vi "ATE_ops_cal_2.vi"() -> ()   [LabVIEW 2009]
doc: "Use this template to build a producer/consumer design pattern with events to produce queue items. Use this design pattern instead of the User Interface Event Handler pattern for user interfaces when you want to execute code asynchronously in response to an event without slowing the user interface responsiveness."
uses:
  Rvp8PowerData.ctl
  <vilib>/Analysis/NI_AALBase.lvlib
  <vilib>/Analysis/NI_AALPro.lvlib
panel:
  in  "ABORT":bool
  in  "READY":bool
  out "Instructions":string="rvp8 calibration vi\n\n1 - Disable or turn off transmitter\n2 - Stow Antenna (point vertically)\n3 - Start the labview program by clicking the Run arrow\n     (left most button under  drop down menues)\n     start cycle time about 35 seconds\n3 - Wait for the red 'BUSY' light to change to green 'READY'\n     The 'active' controls on the control tab are the 'TsPring/TsGrabber'\n     and the 'Start dBm', 'Step Size' and 'Steps' controls \n4 - Calibrate with the red  'Calibrate' button\n      calibration cycle time is about 5 minutes\n5 - Calibration cycle can be aborted with the 'Abort Cal' button which\n     is visable only during the cal cycle\n6 - exit the program with the red 'EXIT' button\n      exit cycle time about 20 seconds\n\nHints:\nWait for the green 'READY' light before clicking buttons"
  out "70dB\nAttenuators":bool[](array[boolean])
  out "70 Verfied":bool
  out "121dB\nAttenuators":bool[](array[boolean])
  out "121 Verified":bool
  in  "Configuration 1":bool
  out "Cal Output File":path
  out "Cal differences":cluster{dbl[], dbl[]}[](graph)
  out "RVP8 calibration":cluster{dbl[], dbl[]}[](graph)
  out "Cal file name":string
  in  "Cal data directory":string="/home/operator/ate/data/rvp8_cal"
  in  "Set SigGen":bool
  in  "Initialize":bool
  in  "70 dB":bool
  in  "121 dB":bool
  in  "Switches":bool
  in  "Calibrate":bool
  in  "Stop":bool
  in  "ATE TABS":enum32{"Status", "Controls"}(tab)=enum."Controls"
  out "ATE Switch Status":T1
  out "RVP8 Power":T2 {"time" format="%<%H:%M:%S\n%Y/%m/%d>T"}
  out "Signal Generator Status":T3={"Frequency (GHz)"=0.0, "RF Power (dBm)"=0.0, "RF Power"=TRUE} {"RF Power (dBm)" format="%.2g"}
  in  "Signal Generator Control":T4={"Frequency (GHz)"=2.809, "RF Power (dBm)"=-120.0, "RF ON/OFF"=FALSE}
  in  "Start dBm":dbl=-14.0 min=-100.0 max=14.0 step=1.0
  in  "Steps":i32=64
  in  "Steps Size":dbl=2.0 min=0.1 max=10.0 step=0.1 format="%.1g"
  in  "121 dB Atten":i32=121 min=0 max=121 step=1
  in  "70 dB Attn":i32=70 min=0 max=70 step=10
  in  "ATE Switches":T5={"Reversing Switch"=enum."Normal Function", "IO Switch #1 Input"=enum."NONE", "IO Switch #1 Output"=enum."NONE", "IO Switch #2 Input"=enum."NONE", "IO Switch #2 Output"=enum."NONE", "Signal Out Input"=enum."NONE", "Signal Out Output"=enum."NONE", "Signal Source Input"=enum."NONE", "Signal Source Output"=enum."NONE", "Power Meter Switch Input"=enum."NONE", "Pouer Meter Switch Output"=enum."NONE", "Amplifier Switch"=enum."Include Amp"}
  in  "DataSource":bool=TRUE
  out "P-State":string
  out "C-State":string
  in  "BUSY":bool
  # "ATE ops cal Program-II"
  # "10 dB"
  # "20 dB"
  # "40 dB"
  # "1 dB"
  # "2 dB"
  # "4 dB"
  # "4 dB"
  # "10 dB"
  # "20 dB"
  # "40 dB"
  # "40 dB"
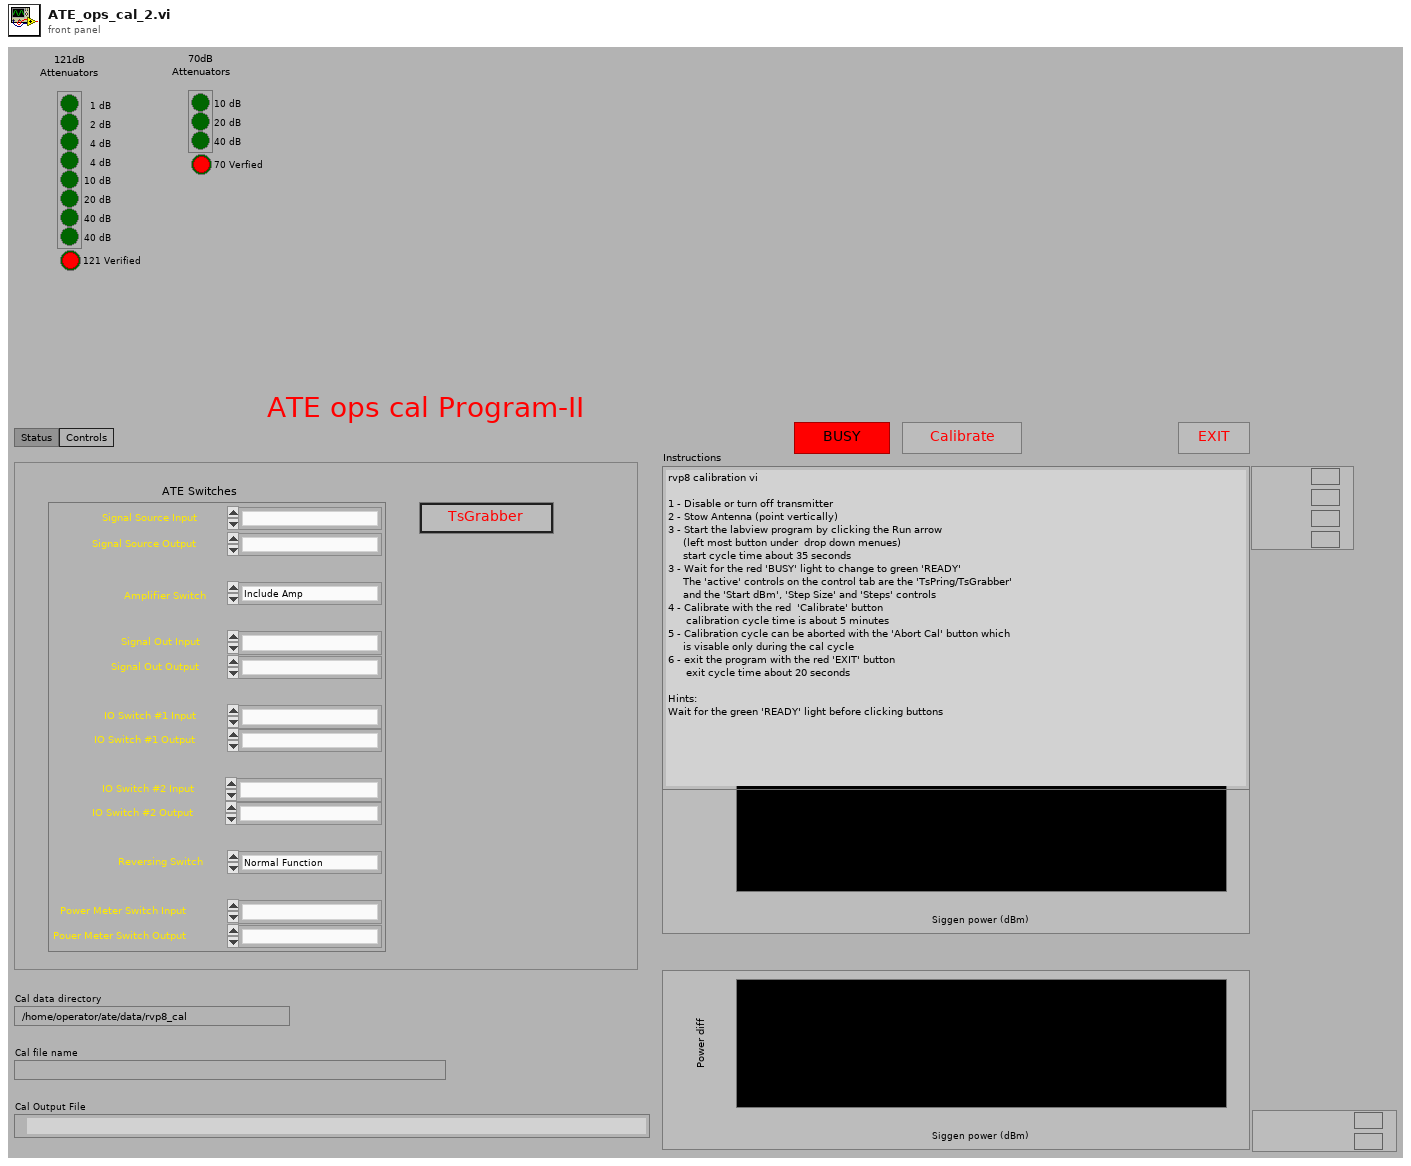
[diagram p1: front panel]
types:
  T1 = cluster{"Reversing Switch ":bool, "IO Switch #1":bool, "IO Switch #2":bool, "Signal Out":bool, "Signal Source":bool, "Power Meter":bool, "Amp By Pass":bool}
  T2 = typedef "Rvp8PowerData.ctl" = cluster{"success":bool, "time":dbl, "el":dbl, "az":dbl, "dbm0":dbl, "dbm1":dbl, "dbmHc":dbl, "dbmHx":dbl, "dbmVc":dbl, "dbmVx":dbl}
  T3 = cluster{"Frequency (GHz)":dbl, "RF Power (dBm)":dbl, "RF Power":bool}
  T4 = cluster{"Frequency (GHz)":dbl, "RF Power (dBm)":dbl, "RF ON/OFF":bool}
  T5 = cluster{"Reversing Switch":enum16{"Normal Function", "Reversing Function"}, "IO Switch #1 Input":enum16{"NONE", "AHR (J2)", "Splitter", "Signal Out Switch (S3)", "Reversing Switch"}, "IO Switch #1 Output":enum16{"NONE", "AHR (J2)", "Delay Device (S4)", "Power Meter Switch (S5)", "Reversing Switch"}, "IO Switch #2 Input":enum16{"NONE", "AVR (J3)", "Splitter", "Signal Out Switch (S3)", " 2W Term (TM1)", "Reversing Switch"}, "IO Switch #2 Output":enum16{"NONE", "AVR (J3)", "Signal Out Switch (S3)", "Power Meter Switch (S5)", "Reversing Switch", "2W Term (TM1)"}, "Signal Out Input":enum16{"NONE", "Amp Bypass Switch (S6)", "IO Switch #1 (S1)", "IO Switch #2 (S2)", "2W Term (TM3)"}, "Signal Out Output":enum16{"NONE", "2 Watt Term (TM3)", "Splitter", "Power Meter Switch (S5)"}, "Signal Source Input":enum16{"NONE", "Delay Device", "Signal Generator (J7)", "Inside Noise Box NF (J5)", "2W Term (TM3)"}, "Signal Source Output":enum16{"NONE", "Amp Bypass Switch", "Test Pulse Generator", "Power Meter Switch (S5)"}, "Power Meter Switch Input":enum16{"NONE", "IO Switch #1 (S1)", "Signal Source Switch (S4)", "Signal Out Switch (S3)", "IO Switch #2 (S2)", "TXH-TXV Switch (J8)"}, "Pouer Meter Switch Output":enum16{"NONE", "Power Meter (J6)"}, "Amplifier Switch":enum16{"Bypass Amp", "Include Amp"}}
  T6 = enum16{"open", "replace", "create", "open or create", "replace or create", "replace or create with confirmation"}
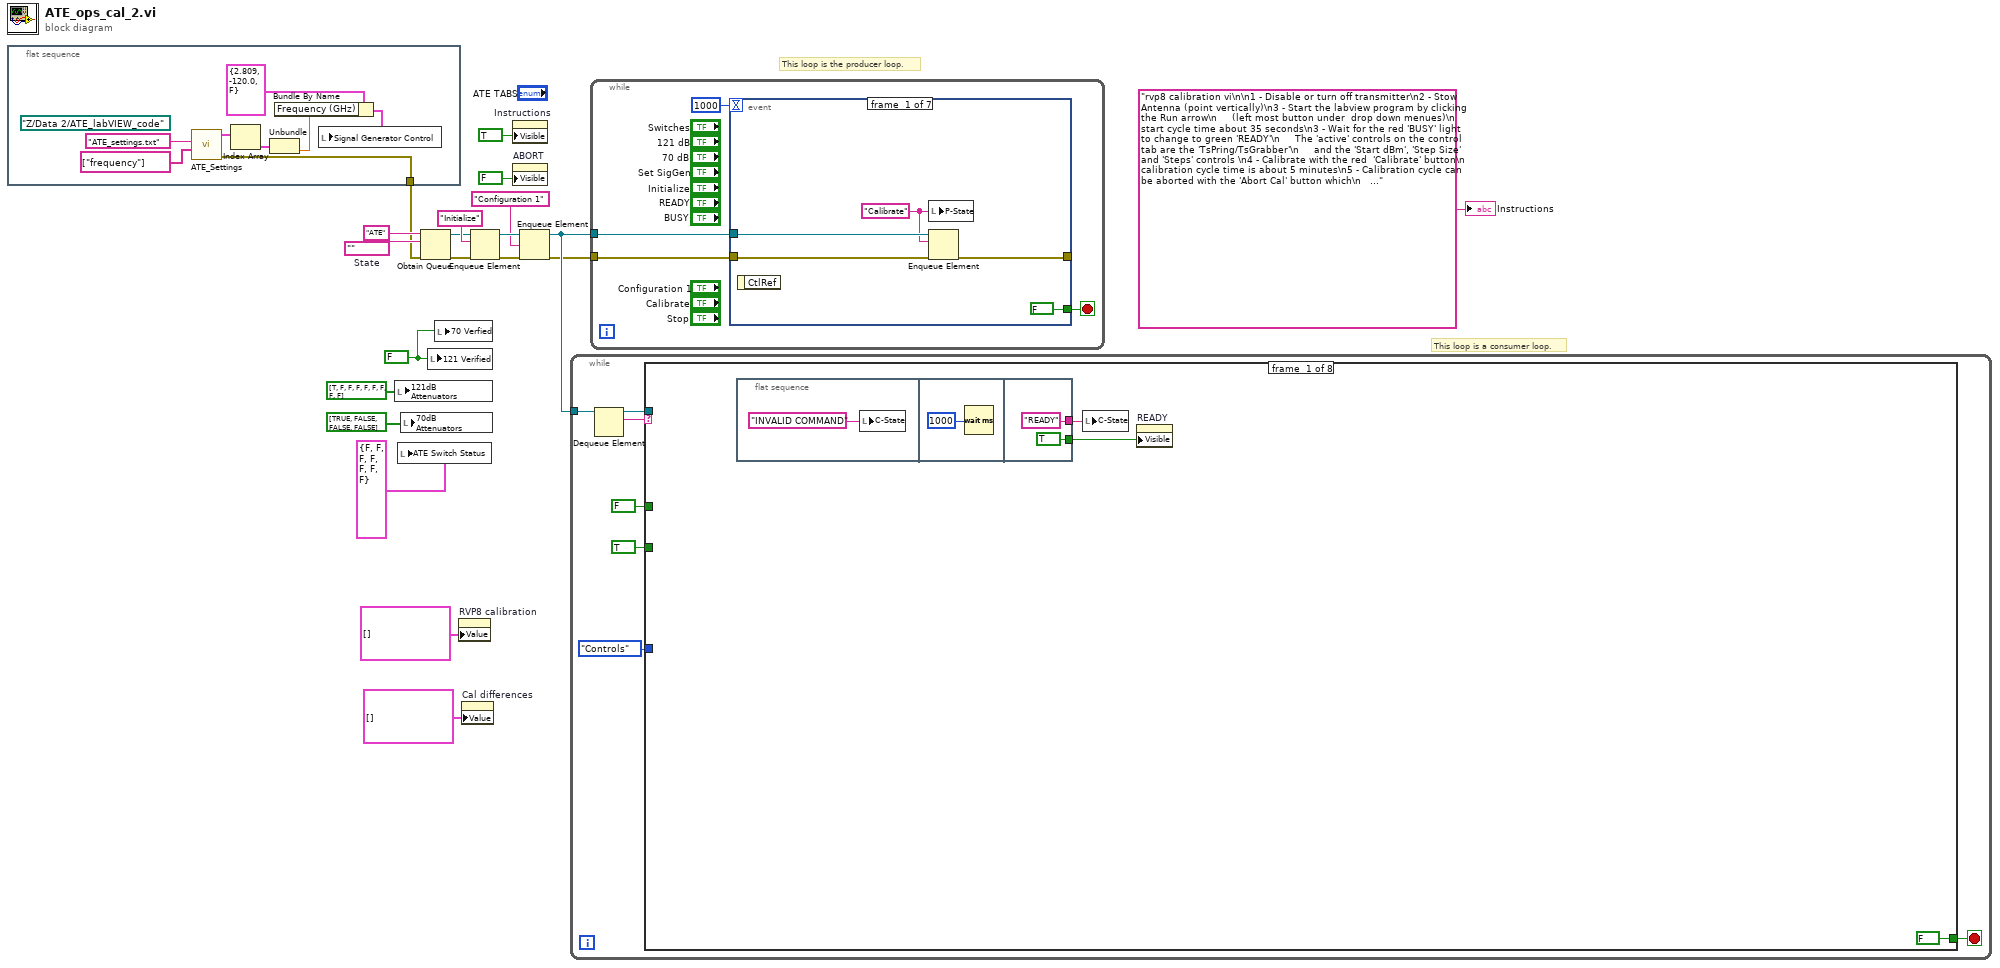
[diagram p0: block diagram]
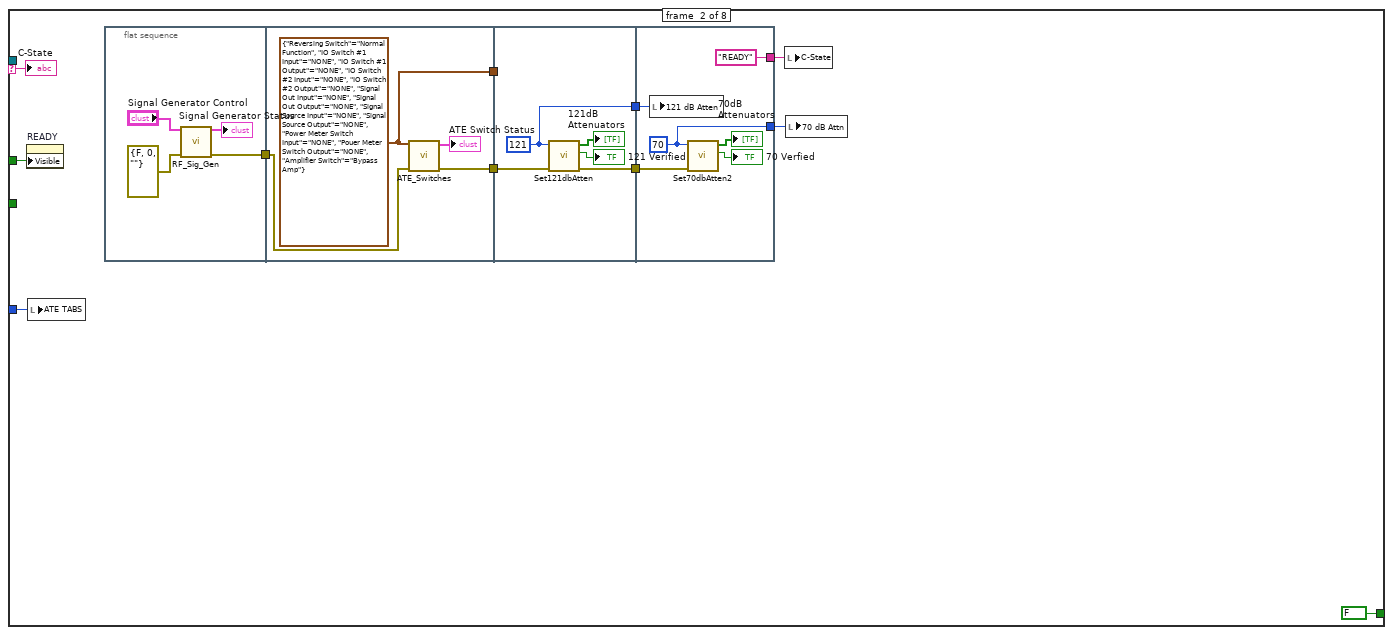
[diagram p2: hidden frame]
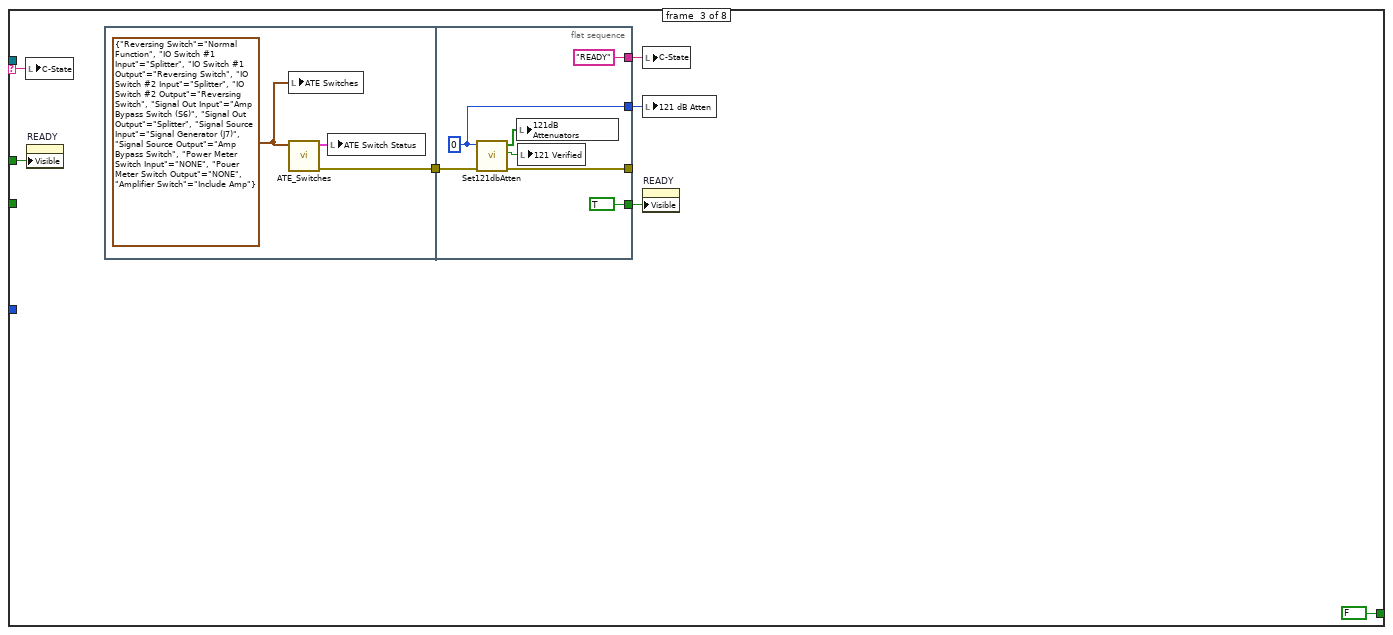
[diagram p3: hidden frame]
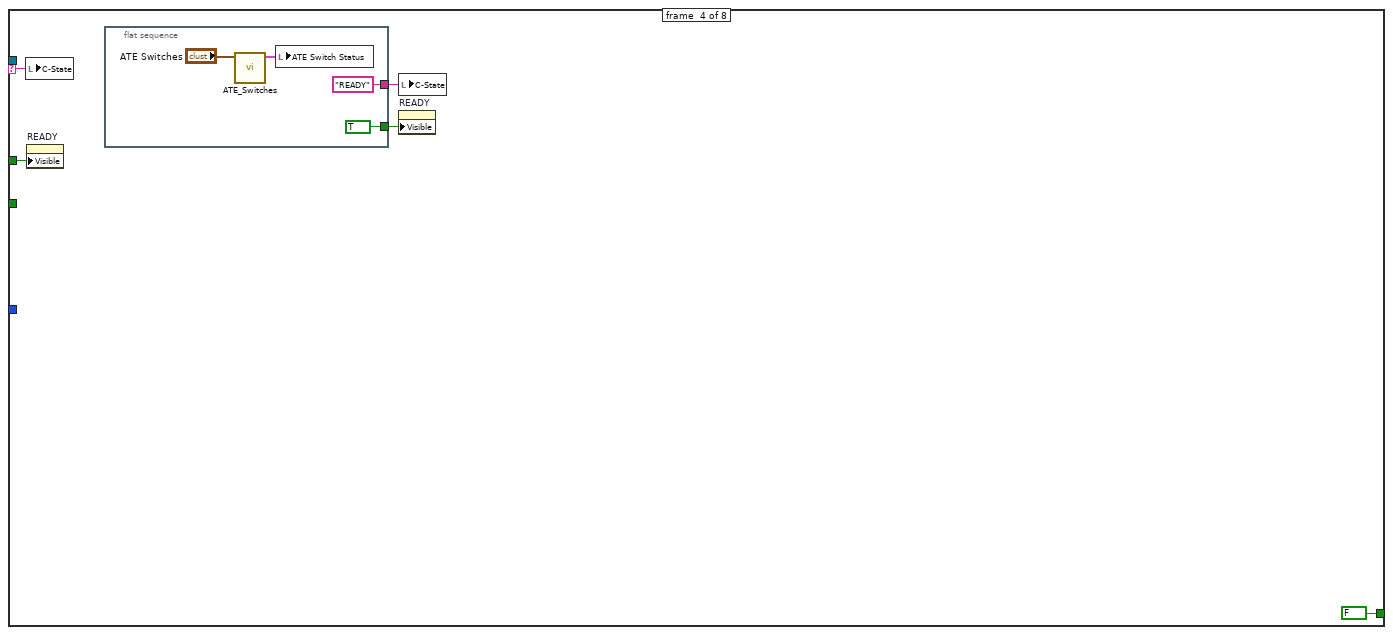
[diagram p4: hidden frame]
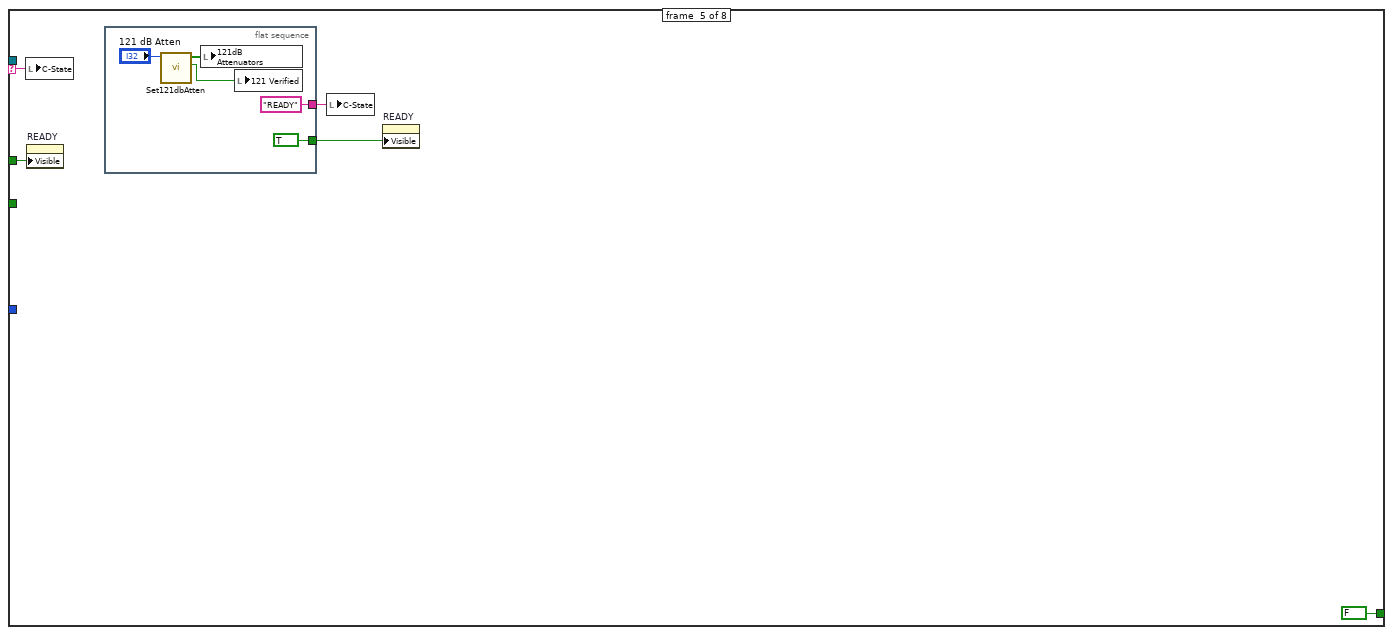
[diagram p5: hidden frame]
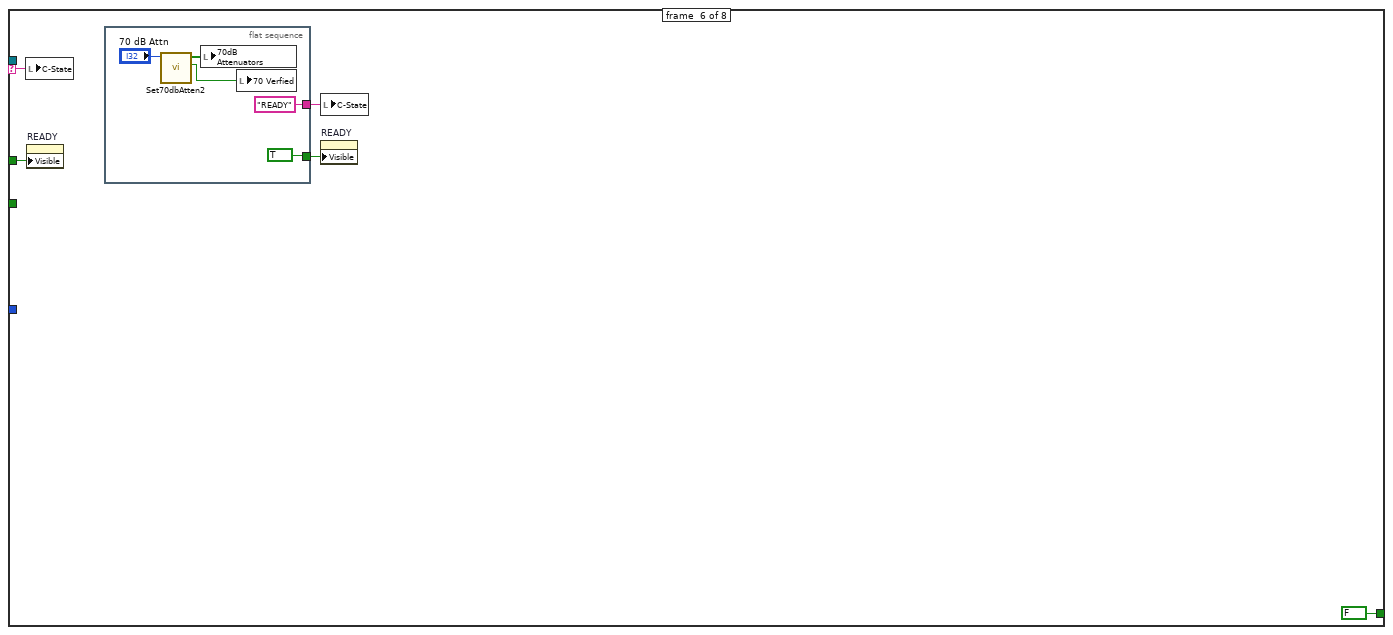
[diagram p6: hidden frame]
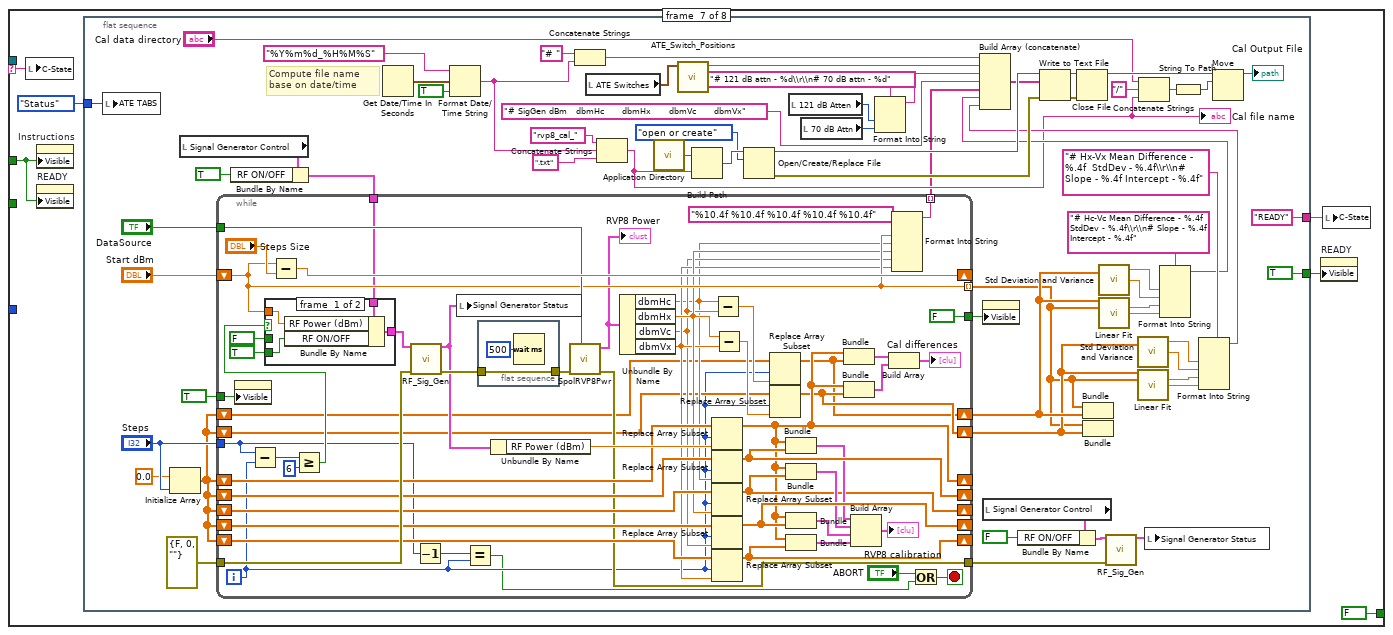
[diagram p7: hidden frame]
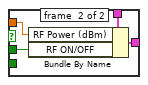
[diagram p8: hidden frame]
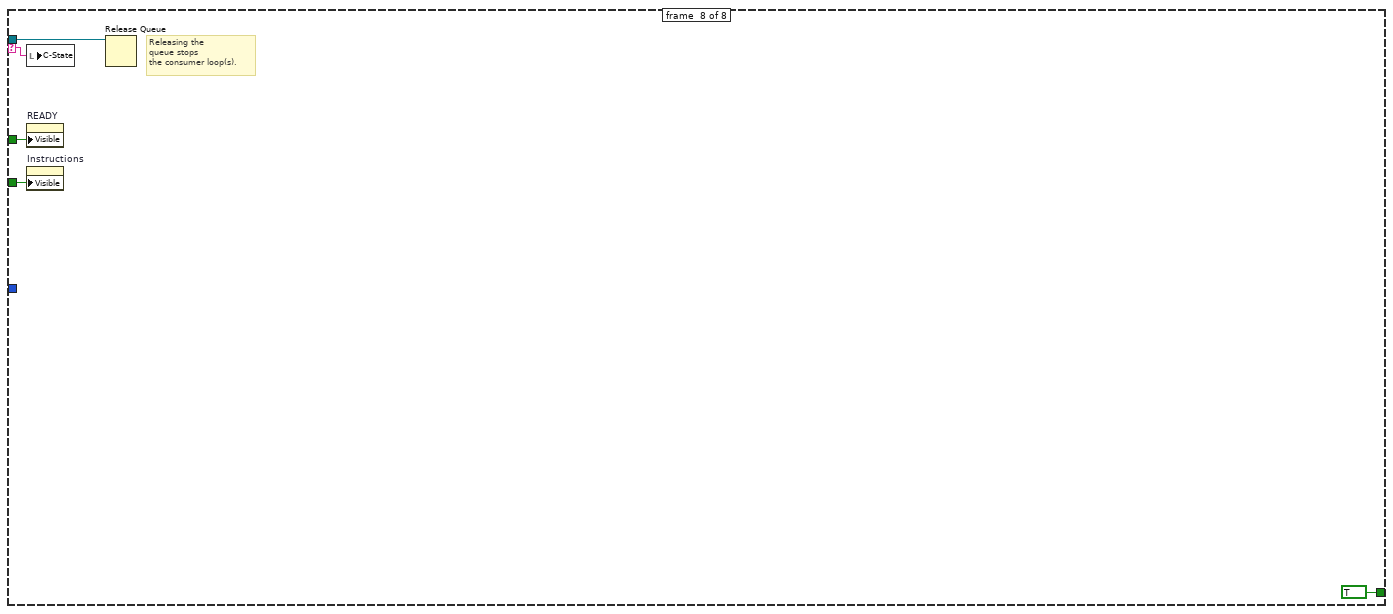
[diagram p9: hidden frame]
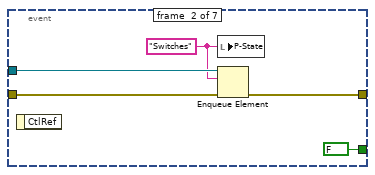
[diagram p10: hidden frame]
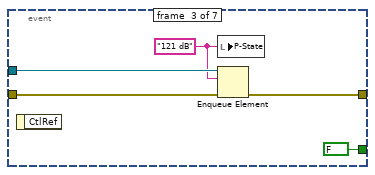
[diagram p11: hidden frame]
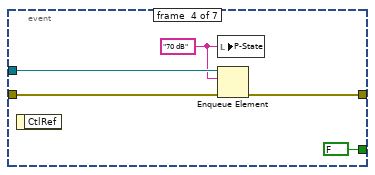
[diagram p12: hidden frame]
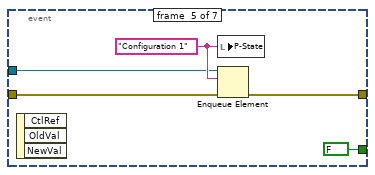
[diagram p13: hidden frame]
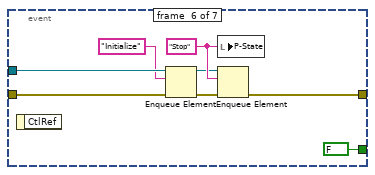
[diagram p14: hidden frame]
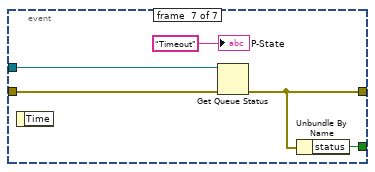
[diagram p15: hidden frame]
diagram:
  w5 = FALSE ("70 Verfied")
  w20 = ""  # State
  # "This loop is the producer loop."
  # "This loop is a consumer loop."
  n1 = flat-sequence {
    tunnel: [w24] -> w1
    frame #0 {
      (unwired) path "Z:/Data 2/ATE_labVIEW_code" ("start path")
      n2 = call "ATE_Settings.vi"("Variable to Read"=string[] ["frequency"], "file name"="ATE_settings.txt") -> ("error out"=w24:errorcluster, "NewVariables"=w26:cluster{"Name":string, "Value":dbl}[])  [unwired: 8 in]
      n3 = Index Array(array=w26) -> (element=w25:cluster{"Name":string, "Value":dbl})  [unwired: 1 in]
      n4 = Unbundle(w25) -> ("Value"=w21:dbl)  [unwired: 1 out]
      n5 = Bundle By Name(cluster=T4 {"Frequency (GHz)"=2.809, "RF Power (dBm)"=-120.0, "RF ON/OFF"=FALSE} ("Signal Generator Control"), "Frequency (GHz)"=w21) -> (w23:T4)
      n6 = local write "Signal Generator Control"(w23) -> ()
    }
  }
  n7 = local write "121dB\nAttenuators"(bool[] [TRUE, FALSE, FALSE, FALSE, FALSE, FALSE, FALSE, FALSE, FALSE] ("121dB\nAttenuators")) -> ()
  n8 = local write "ATE Switch Status"(T1 {"Reversing Switch "=FALSE, "IO Switch #1"=FALSE, "IO Switch #2"=FALSE, "Signal Out"=FALSE, "Signal Source"=FALSE, "Power Meter"=FALSE, "Amp By Pass"=FALSE} ("ATE Switch Status")) -> ()
  n9 = local write "70dB\nAttenuators"(bool[] [TRUE, FALSE, FALSE, FALSE] ("70dB\nAttenuators")) -> ()
  n10 = Obtain Queue(name (unnamed)="ATE", element data type=w20, error in (no error)=w1) -> (queue out=w17:refnum<queue>, error out=w15:errorcluster)  [unwired: 2 in, 1 out]
  n11 = local write "121 Verified"(w5) -> ()
  n12 = local write "70 Verfied"(w5) -> ()
  n13 = property on="RVP8 calibration" class="XYGraph (strict)"("Value"=cluster{dbl[], dbl[]}[] [] ("RVP8 calibration")) -> ()  [unwired: 2 in, 2 out]
  n14 = property on="Cal differences" class="XYGraph (strict)"("Value"=cluster{dbl[], dbl[]}[] [] ("Cal differences")) -> ()  [unwired: 2 in, 2 out]
  n15 = Enqueue Element(queue=w17, element="Initialize", error in (no error)=w15) -> (queue out=w16:refnum<queue>, error out=w10:errorcluster)  [unwired: 1 in, 1 out]
  n16 = property on="Instructions" class="Str"("Visible"=TRUE) -> ()  [unwired: 2 in, 2 out]
  n17 = property on="ABORT" class="Bool"("Visible"=FALSE) -> ()  [unwired: 2 in, 2 out]
  n18 = Enqueue Element(queue=w16, element="Configuration 1", error in (no error)=w10) -> (queue out=w11:refnum<queue>, error out=w9:errorcluster)  [unwired: 1 in, 1 out]
  n19 = while {
    tunnel: w11 -> [w35]
    stop <- w32 stop-if-true
    n20 = Dequeue Element(queue=w35) -> (queue out=w33:refnum<queue>, element=w34:string)  [unwired: 2 in, 2 out]
    n21 = case shown="\"Initialize\"" w34 {
      selector: w34 -> [_ w52 w75 w94 w102 w112 w123 w259]
      tunnel: w33 -> [_ _ _ _ _ _ _ w258]
      tunnel: [FALSE FALSE FALSE FALSE FALSE FALSE FALSE TRUE] -> w32
      tunnel: FALSE ("Visible") -> [_ w44 w74 w91 w100 w110 w121 w257]
      tunnel: TRUE ("Visible") -> [_ _ _ _ _ _ _ w256]
      tunnel: enum32{"Status", "Controls"}."Controls" ("ATE TABS") -> [_ w43 _ _ _ _ _ _]
      frame #0 {
        n22 = flat-sequence {
          tunnel: ["READY" ("element")] -> w37
          tunnel: [TRUE ("Visible")] -> w36
          frame #0 {
            n23 = local write "C-State"("INVALID COMMAND" ("C-State")) -> ()
          }
          frame #1 {
            n24 = Wait (ms)(milliseconds to wait=u32 1000) -> ()  [unwired: 1 out]
          }
          frame #2 {
          }
        }
        n25 = local write "C-State"(w37) -> ()
        n26 = property on="READY" class="Bool"("Visible"=w36) -> ()  [unwired: 2 in, 2 out]
      }
      frame #1 {
        n27 = property on="READY" class="Bool"("Visible"=w44) -> ()  [unwired: 2 in, 2 out]
        n28 = local write "ATE TABS"(w43) -> ()
        n29 = flat-sequence {
          tunnel: [w54] -> w46
          tunnel: [w59] -> w49
          tunnel: w46 -> [w60]
          tunnel: [w58] -> w45
          tunnel: w49 -> [w65]
          tunnel: [w64] -> w50
          tunnel: [w63] -> w48
          tunnel: w45 -> [_]
          tunnel: ["READY" ("element")] -> w51
          tunnel: w50 -> [w71]
          tunnel: w48 -> [w69]
          tunnel: [w68] -> w47
          frame #0 {
            n30 = call "RF_Sig_Gen.vi"("Signal Generator Control"="Signal Generator Control", "error in"=errorcluster {"status"=FALSE, "code"=0, "source"=""}) -> ("Signal Generator Status"=→"Signal Generator Status":T3, "Sig Gen Errors"=w54:errorcluster)  [unwired: 12 in]
          }
          frame #1 {
            w58 = T5 {"Reversing Switch"=enum."Normal Function", "IO Switch #1 Input"=enum."NONE", "IO Switch #1 Output"=enum."NONE", "IO Switch #2 Input"=enum."NONE", "IO Switch #2 Output"=enum."NONE", "Signal Out Input"=enum."NONE", "Signal Out Output"=enum."NONE", "Signal Source Input"=enum."NONE", "Signal Source Output"=enum."NONE", "Power Meter Switch Input"=enum."NONE", "Pouer Meter Switch Output"=enum."NONE", "Amplifier Switch"=enum."Bypass Amp"} ("ATE Switches")
            n31 = call "ATE_Switches.vi"("error in"=w60, "ATE Switches"=w58) -> ("Switch Errors"=w59:errorcluster, "ATE Switch Status"=→"ATE Switch Status":T1)  [unwired: 8 in]
          }
          frame #2 {
            w63 = 121 ("Attenuation (dB)")
            n32 = call "Set121dbAtten.vi"("error in (no error)"=w65, "Attenuation (dB)"=w63) -> ("error out"=w64:errorcluster, "Verfied"=→"121 Verified":bool, "Active Attenuators"=→"121dB\nAttenuators":bool[])  [unwired: 7 in]
          }
          frame #3 {
            w68 = 70 ("Attenuation (dB)")
            n33 = local write "121 dB Atten"(w69) -> ()
            n34 = call "Set70dbAtten2.vi"("error in (no error)"=w71, "Attenuation (dB)"=w68) -> ("Verfied"=→"70 Verfied":bool, "Active Attenuators"=→"70dB\nAttenuators":bool[])  [unwired: 7 in, 1 out]
          }
        }
        n35 = local write "C-State"(w51) -> ()
        n36 = local write "70 dB Attn"(w47) -> ()
        "C-State" <- w52
      }
      frame #2 {
        n37 = local write "C-State"(w75) -> ()
        n38 = property on="READY" class="Bool"("Visible"=w74) -> ()  [unwired: 2 in, 2 out]
        n39 = flat-sequence {
          tunnel: [w82] -> w78
          tunnel: w78 -> [w89]
          tunnel: [w84] -> w77
          tunnel: ["READY" ("element")] -> w76
          tunnel: [w87] -> _
          tunnel: [TRUE ("Visible")] -> w73
          frame #0 {
            w80 = T5 {"Reversing Switch"=enum."Normal Function", "IO Switch #1 Input"=enum."Splitter", "IO Switch #1 Output"=enum."Reversing Switch", "IO Switch #2 Input"=enum."Splitter", "IO Switch #2 Output"=enum."Reversing Switch", "Signal Out Input"=enum."Amp Bypass Switch (S6)", "Signal Out Output"=enum."Splitter", "Signal Source Input"=enum."Signal Generator (J7)", "Signal Source Output"=enum."Amp Bypass Switch", "Power Meter Switch Input"=enum."NONE", "Pouer Meter Switch Output"=enum."NONE", "Amplifier Switch"=enum."Include Amp"} ("ATE Switches")
            n40 = local write "ATE Switches"(w80) -> ()
            n41 = call "ATE_Switches.vi"("ATE Switches"=w80) -> ("Switch Errors"=w82:errorcluster, "ATE Switch Status"=w81:T1)  [unwired: 9 in]
            n42 = local write "ATE Switch Status"(w81) -> ()
          }
          frame #1 {
            w84 = 0 ("Attenuation (dB)")
            n43 = call "Set121dbAtten.vi"("error in (no error)"=w89, "Attenuation (dB)"=w84) -> ("error out"=w87:errorcluster, "Verfied"=w85:bool, "Active Attenuators"=w86:bool[])  [unwired: 7 in]
            n44 = local write "121dB\nAttenuators"(w86) -> ()
            n45 = local write "121 Verified"(w85) -> ()
          }
        }
        n46 = local write "C-State"(w76) -> ()
        n47 = local write "121 dB Atten"(w77) -> ()
        n48 = property on="READY" class="Bool"("Visible"=w73) -> ()  [unwired: 2 in, 2 out]
      }
      frame #3 {
        n49 = local write "C-State"(w94) -> ()
        n50 = property on="READY" class="Bool"("Visible"=w91) -> ()  [unwired: 2 in, 2 out]
        n51 = flat-sequence {
          tunnel: ["READY" ("element")] -> w92
          tunnel: [TRUE ("Visible")] -> w90
          frame #0 {
            n52 = call "ATE_Switches.vi"("ATE Switches"="ATE Switches") -> ("ATE Switch Status"=w97:T1)  [unwired: 9 in, 1 out]
            n53 = local write "ATE Switch Status"(w97) -> ()
          }
        }
        n54 = local write "C-State"(w92) -> ()
        n55 = property on="READY" class="Bool"("Visible"=w90) -> ()  [unwired: 2 in, 2 out]
      }
      frame #4 {
        n56 = local write "C-State"(w102) -> ()
        n57 = property on="READY" class="Bool"("Visible"=w100) -> ()  [unwired: 2 in, 2 out]
        n58 = flat-sequence {
          tunnel: ["READY" ("element")] -> w101
          tunnel: [TRUE ("Visible")] -> w99
          frame #0 {
            n59 = call "Set121dbAtten.vi"("Attenuation (dB)"="121 dB Atten") -> ("Verfied"=w105:bool, "Active Attenuators"=w107:bool[])  [unwired: 8 in, 1 out]
            n60 = local write "121dB\nAttenuators"(w107) -> ()
            n61 = local write "121 Verified"(w105) -> ()
          }
        }
        n62 = local write "C-State"(w101) -> ()
        n63 = property on="READY" class="Bool"("Visible"=w99) -> ()  [unwired: 2 in, 2 out]
      }
      frame #5 {
        n64 = local write "C-State"(w112) -> ()
        n65 = property on="READY" class="Bool"("Visible"=w110) -> ()  [unwired: 2 in, 2 out]
        n66 = flat-sequence {
          tunnel: ["READY" ("element")] -> w111
          tunnel: [TRUE ("Visible")] -> w109
          frame #0 {
            n67 = call "Set70dbAtten2.vi"("Attenuation (dB)"="70 dB Attn") -> ("Verfied"=w115:bool, "Active Attenuators"=w117:bool[])  [unwired: 8 in, 1 out]
            n68 = local write "70dB\nAttenuators"(w117) -> ()
            n69 = local write "70 Verfied"(w115) -> ()
          }
        }
        n70 = local write "C-State"(w111) -> ()
        n71 = property on="READY" class="Bool"("Visible"=w109) -> ()  [unwired: 2 in, 2 out]
      }
      frame #6 {
        n72 = local write "C-State"(w123) -> ()
        n73 = property on="Instructions" class="Str"("Visible"=w121) -> ()  [unwired: 2 in, 2 out]
        n74 = property on="READY" class="Bool"("Visible"=w121) -> ()  [unwired: 2 in, 2 out]
        n75 = flat-sequence {
          tunnel: ["READY" ("element")] -> w122
          tunnel: [TRUE ("Visible")] -> w120
          tunnel: enum32{"Status", "Controls"}."Status" ("ATE TABS") -> [w134]
          frame #0 {
            # "Compute file name base on date/time"
            n76 = local write "ATE TABS"(w134) -> ()
            n77 = Initialize Array(0.0 ("element"), "Steps") -> (w133:dbl[])
            n78 = local read "Signal Generator Control"() -> (w129:T4)
            n79 = Bundle By Name(cluster=w129, "RF ON/OFF"=TRUE) -> (w128:T4)
            n80 = while {
              shift-right: [w240] -> _
              shift-left: "Start dBm" -> [w237]
              tunnel: errorcluster {"status"=FALSE, "code"=0, "source"=""} ("error out") -> [w231]
              tunnel: [w237] -> w136 mode=indexing
              tunnel: [w245] -> w139 mode=indexing
              tunnel: [w209] -> w171
              tunnel: "DataSource" -> [w239]
              tunnel: "Steps" -> [w194]
              shift-right: [w208] -> _
              shift-left: w133 -> [w223]
              shift-right: [w220] -> _
              shift-left: w133 -> [w227]
              shift-right: [w210] -> _
              shift-left: w133 -> [w228]
              shift-right: [w222] -> _
              shift-left: w133 -> [w229]
              shift-right: [w221] -> _
              shift-left: w133 -> [w230]
              shift-right: [w204] -> w162
              shift-left: w133 -> [w202]
              shift-right: [w205] -> w161
              shift-left: w133 -> [w203]
              tunnel: [FALSE ("Visible")] -> w132
              tunnel: TRUE ("Visible") -> [w191]
              tunnel: w128 -> [w190]
              i -> [w196]
              stop <- w198 stop-if-true
              n81 = property on="ABORT" class="Bool"("Visible"=w191) -> ()  [unwired: 2 in, 2 out]
              n82 = Subtract(x=w194, y=w196) -> (x-y=w232:i32)
              n83 = Subtract(x=w237, y="Steps Size") -> (x-y=w240:dbl)
              n84 = Greater Or Equal?(x=w232, y=6) -> (x >= y?=w234:bool)
              n85 = case shown="False" w234 {
                tunnel: w190 -> [w249 w253]
                tunnel: [w248 w252] -> w241
                tunnel: w237 -> [w247 w251]
                tunnel: FALSE ("70 Verfied") -> [_ w250]
                tunnel: TRUE ("70 Verfied") -> [w246 _]
                frame #0 {
                  n86 = Bundle By Name(cluster=w249, "RF Power (dBm)"=w247, "RF ON/OFF"=w246) -> (w248:T4)
                }
                frame #1 {
                  n87 = Bundle By Name(cluster=w253, "RF Power (dBm)"=w251, "RF ON/OFF"=w250) -> (w252:T4)
                }
              }
              n88 = call "RF_Sig_Gen.vi"("Signal Generator Control"=w241, "error in"=w231) -> ("Signal Generator Status"=w225:T3, "Sig Gen Errors"=w244:errorcluster)  [unwired: 12 in]
              n89 = Decrement(x=w194) -> (x-1=w195:i32)
              n90 = local write "Signal Generator Status"(w225) -> ()
              n91 = Equal?(x=w195, y=w196) -> (x = y?=w193:bool)
              n92 = flat-sequence {
                tunnel: w244 -> [w255]
                tunnel: [w255] -> w243
                frame #0 {
                  n93 = Wait (ms)(milliseconds to wait=u32 500) -> ()  [unwired: 1 out]
                }
              }
              n94 = Unbundle By Name(w225) -> ("RF Power (dBm)"=w224:dbl)
              n95 = call "SpolRVP8Pwr.vi"("DataSource"=w239, "error in (no error)"=w243) -> ("Comm error"=w209:errorcluster, "RVP8_power"=w226:T2)  [unwired: 6 in, 2 out]
              "RVP8 Power" <- w226
              n96 = Unbundle By Name(w226) -> ("dbmHc"=w211:dbl, "dbmHx"=w214:dbl, "dbmVc"=w212:dbl, "dbmVx"=w213:dbl)
              n97 = Replace Array Subset(array=w223, new element=w224, index=w196) -> (w208:dbl[])
              n98 = Replace Array Subset(array=w227, new element=w211, index=w196) -> (w220:dbl[])
              n99 = Replace Array Subset(array=w228, new element=w214, index=w196) -> (w210:dbl[])
              n100 = Replace Array Subset(array=w229, new element=w212, index=w196) -> (w222:dbl[])
              n101 = Replace Array Subset(array=w230, new element=w213, index=w196) -> (w221:dbl[])
              n102 = Subtract(x=w211, y=w212) -> (x-y=w207:dbl)
              n103 = Subtract(x=w214, y=w213) -> (x-y=w206:dbl)
              n104 = Replace Array Subset(array=w202, new element=w207, index=w196) -> (w204:dbl[])
              n105 = Replace Array Subset(array=w203, new element=w206, index=w196) -> (w205:dbl[])
              n106 = Bundle(w208, w220) -> (w216:cluster{dbl[], dbl[]})  [unwired: 1 in]
              n107 = Bundle(w208, w210) -> (w217:cluster{dbl[], dbl[]})  [unwired: 1 in]
              n108 = Bundle(w208, w222) -> (w218:cluster{dbl[], dbl[]})  [unwired: 1 in]
              n109 = Bundle(w208, w221) -> (w219:cluster{dbl[], dbl[]})  [unwired: 1 in]
              n110 = Bundle(w208, w204) -> (w200:cluster{dbl[], dbl[]})  [unwired: 1 in]
              n111 = Bundle(w208, w205) -> (w201:cluster{dbl[], dbl[]})  [unwired: 1 in]
              n112 = Build Array(w216, w217, w218, w219) -> (→"RVP8 calibration":cluster{dbl[], dbl[]}[])
              n113 = Build Array(w200, w201) -> (→"Cal differences":cluster{dbl[], dbl[]}[])
              n114 = Format Into String(format string="%10.4f %10.4f %10.4f %10.4f %10.4f", w237, w211, w214, w212, w213) -> (resulting string=w245:string)  [unwired: 2 in, 1 out]
              n115 = Or(x="ABORT", y=w193) -> (x .or. y?=w198:bool)
            }
            n116 = Get Date/Time In Seconds() -> (seconds since 1Jan1904=w184:timestamp)
            n117 = Format Date/Time String(time format string (%c)="%Y%m%d_%H%M%S", seconds (now)=w184, UTC format=TRUE) -> (date/time string=w141:string)
            n118 = Concatenate Strings("# " ("string"), w141) -> (w154:string)
            n119 = local read "ATE Switches"() -> (w148:T5)
            n120 = Concatenate Strings("rvp8_cal_", w141, ".txt") -> (w140:string)
            "Cal file name" <- w140
            n121 = call <vilib>:"Application Directory.vi"() -> ("Application Directory"=w145:path)
            n122 = call "ATE_Switch_Positions.vi"("ATE Switches"=w148) -> ("ATE Switch/Position"=w153:string)  [unwired: 10 in]
            n123 = Build Path(base path=w145, name or relative path=w140) -> (appended path=w182:path)
            n124 = Open/Create/Replace File(file path (use dialog)=w182, operation (0:open)=T6."open or create") -> (refnum out=w181:refnum<file>, error out=w180:errorcluster)  [unwired: 4 in, 1 out]
            n125 = local read "121 dB Atten"() -> (w168:i32)
            n126 = local read "70 dB Attn"() -> (w167:i32)
            n127 = Format Into String(format string="# 121 dB attn - %d\\r\\n# 70 dB attn - %d", w168, w167) -> (resulting string=w152:string)  [unwired: 2 in, 1 out]
            n128 = property on="ABORT" class="Bool"("Visible"=w132) -> ()  [unwired: 2 in, 2 out]
            n129 = local read "Signal Generator Control"() -> (w126:T4)
            n130 = Bundle By Name(cluster=w126, "RF ON/OFF"=FALSE) -> (w125:T4)
            n131 = Bundle(w136, w162) -> ()  [unwired: 1 in, 1 out]
            n132 = Bundle(w136, w161) -> ()  [unwired: 1 in, 1 out]
            n133 = call <vilib>:"Std Deviation and Variance.vi"("X"=w162) -> ("mean"=w166:dbl, "standard deviation"=w163:dbl)  [unwired: 1 in, 1 out]
            n134 = call <vilib>:"Linear Fit.vi"("Y"=w162, "X"=w136) -> ("slope"=w165:dbl, "intercept"=w164:dbl)  [unwired: 9 in, 3 out]
            n135 = call "RF_Sig_Gen.vi"("Signal Generator Control"=w125, "error in"=w171) -> ("Signal Generator Status"=w172:T3)  [unwired: 12 in, 1 out]
            n136 = call <vilib>:"Std Deviation and Variance.vi"("X"=w161) -> ("mean"=w160:dbl, "standard deviation"=w159:dbl)  [unwired: 1 in, 1 out]
            n137 = call <vilib>:"Linear Fit.vi"("Y"=w161, "X"=w136) -> ("slope"=w158:dbl, "intercept"=w157:dbl)  [unwired: 9 in, 3 out]
            n138 = Concatenate Strings("Cal data directory", "/" ("string"), w140) -> (w176:string)
            n139 = local write "Signal Generator Status"(w172) -> ()
            n140 = Format Into String(format string="# Hc-Vc Mean Difference - %.4f  StdDev - %.4f\\r\\n# Slope - %.4f Intercept - %.4f", w166, w163, w165, w164) -> (resulting string=w144:string)  [unwired: 2 in, 1 out]
            n141 = String To Path(string=w176) -> (path=w174:path)
            n142 = Format Into String(format string="# Hx-Vx Mean Difference - %.4f  StdDev - %.4f\\r\\n# Slope - %.4f Intercept - %.4f", w160, w159, w158, w157) -> (resulting string=w143:string)  [unwired: 2 in, 1 out]
            n143 = Build Array (concatenate)(w154, w153, w152, "# SigGen dBm   dbmHc      dbmHx      dbmVc      dbmVx", w139, w144, w143) -> (w170:string[])
            n144 = Write to Text File(file (use dialog)=w181, text=w170, error in=w180) -> (refnum out=w179:refnum<file>, error out=w178:errorcluster)  [unwired: 1 in, 1 out]
            n145 = Close File(refnum=w179, error in=w178) -> (path=w175:path)  [unwired: 1 out]
            n146 = Move(source path=w175, 10:w174) -> (3:→"Cal Output File":path)  [unwired: 3 in, 2 out]
          }
        }
        n147 = property on="READY" class="Bool"("Visible"=w120) -> ()  [unwired: 2 in, 2 out]
        n148 = local write "C-State"(w122) -> ()
      }
      frame #7 {
        # "Releasing the\nqueue stops\nthe consumer loop(s)."
        n149 = local write "C-State"(w259) -> ()
        n150 = property on="READY" class="Bool"("Visible"=w257) -> ()  [unwired: 2 in, 2 out]
        n151 = property on="Instructions" class="Str"("Visible"=w256) -> ()  [unwired: 2 in, 2 out]
        n152 = Release Queue(queue=w258) -> ()  [unwired: 2 in, 3 out]
      }
    }
  }
  n153 = while {
    tunnel: w11 -> [w264]
    tunnel: w9 -> [w263]
    stop <- w261 stop-if-true
    n154 = event shown="[4] \"Configuration 1\": Value Change" {
      selector: _ -> [_ _ _ _ _ _ _]
      dyn-events: _ -> [_ _ _ _ _ _ _]
      timeout: 1000 -> [_ _ _ _ _ _ _]
      tunnel: w264 -> [w269 w274 w279 w284 w288 w292 w302]
      tunnel: w263 -> [w268 w273 w278 w283 w287 w294 w298]
      tunnel: [w267 w272 w277 w282 w286 w297 w300] -> _
      tunnel: [FALSE FALSE FALSE FALSE FALSE ("status") FALSE w301] -> w261
      event #0 {
        w265 = "Calibrate" ("element")
        n155 = event-data() -> ()  [unwired: 1 in, 1 out]
        n156 = local write "P-State"(w265) -> ()
        n157 = Enqueue Element(queue=w269, element=w265, error in (no error)=w268) -> (error out=w267:errorcluster)  [unwired: 1 in, 2 out]
      }
      event #1 {
        w270 = "Switches" ("element")
        n158 = event-data() -> ()  [unwired: 1 in, 1 out]
        n159 = local write "P-State"(w270) -> ()
        n160 = Enqueue Element(queue=w274, element=w270, error in (no error)=w273) -> (error out=w272:errorcluster)  [unwired: 1 in, 2 out]
      }
      event #2 {
        w275 = "121 dB" ("element")
        n161 = event-data() -> ()  [unwired: 1 in, 1 out]
        n162 = local write "P-State"(w275) -> ()
        n163 = Enqueue Element(queue=w279, element=w275, error in (no error)=w278) -> (error out=w277:errorcluster)  [unwired: 1 in, 2 out]
      }
      event #3 {
        w280 = "70 dB" ("element")
        n164 = event-data() -> ()  [unwired: 1 in, 1 out]
        n165 = local write "P-State"(w280) -> ()
        n166 = Enqueue Element(queue=w284, element=w280, error in (no error)=w283) -> (error out=w282:errorcluster)  [unwired: 1 in, 2 out]
      }
      event #4 {
        w289 = "Configuration 1" ("element")
        n167 = event-data() -> ()  [unwired: 1 in, 3 out]
        n168 = local write "P-State"(w289) -> ()
        n169 = Enqueue Element(queue=w288, element=w289, error in (no error)=w287) -> (error out=w286:errorcluster)  [unwired: 1 in, 2 out]
      }
      event #5 {
        w295 = "Stop" ("element")
        n170 = event-data() -> ()  [unwired: 1 in, 1 out]
        n171 = Enqueue Element(queue=w292, element="Initialize", error in (no error)=w294) -> (queue out=w291:refnum<queue>, error out=w293:errorcluster)  [unwired: 1 in, 1 out]
        n172 = local write "P-State"(w295) -> ()
        n173 = Enqueue Element(queue=w291, element=w295, error in (no error)=w293) -> (error out=w297:errorcluster)  [unwired: 1 in, 2 out]
      }
      event #6 {
        n174 = event-data() -> ()  [unwired: 1 in, 1 out]
        n175 = Get Queue Status(queue=w302, error in (no error)=w298) -> (error out=w300:errorcluster)  [unwired: 1 in, 7 out]
        n176 = Unbundle By Name(w300) -> ("status"=w301:bool)
        "P-State" <- "Timeout" ("element")
      }
    }
  }
  "Instructions" <- "rvp8 calibration vi\n\n1 - Disable or turn off transmitter\n2 - Stow Antenna (point vertically)\n3 - Start the labview program by clicking the Run arrow\n     (left most button under  drop down menues)\n     start cycle time about 35 seconds\n3 - Wait for the red 'BUSY' light to change to green 'READY'\n     The 'active' controls on the control tab are the 'TsPring/TsGrabber'\n     and the 'Start dBm', 'Step Size' and 'Steps' controls \n4 - Calibrate with the red  'Calibrate' button\n      calibration cycle time is about 5 minutes\n5 - Calibration cycle can be aborted with the 'Abort Cal' button which\n     is visable only during the cal cycle\n6 - exit the program with the red 'EXIT' button\n      exit cycle time about 20 seconds\n\nHints:\nWait for the green 'READY' light before clicking buttons" ("String")
